vi "Read Debug Data Event.vi"(8 "error in (no error)":errorcluster, 11 "Debug Message Receiver In":refnum<class "Mock Debug Message Receiver.lvclass">) -> (0 "error out":errorcluster, 2 "Debug Data Event":refnum<user-event>, 3 "Debug Message Receiver Out":refnum<class "Mock Debug Message Receiver.lvclass">)   [LabVIEW 2020, in "Mock Debug Message Receiver.lvclass"]
uses:
  Mock Debug Message Receiver.lvclass
  Debug Message Receiver/Public/Debug Data Cluster.ctl
  Mock Debug Message Receiver.lvclass/Mock Debug Message Receiver.ctl
  Debug Data Event/Debug Data Event.lvclass
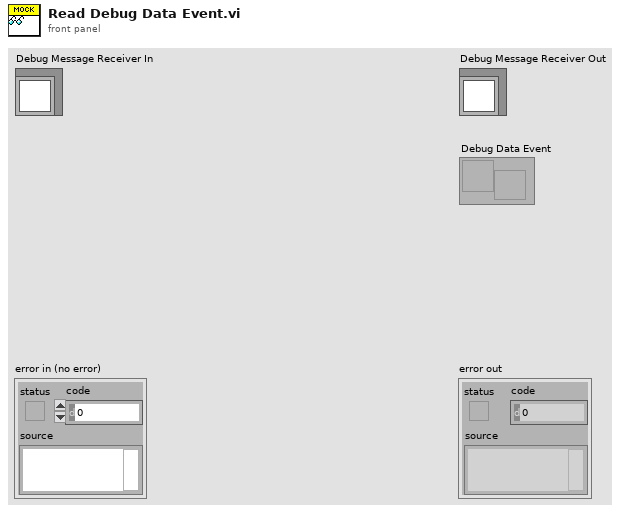
[diagram p1: front panel]
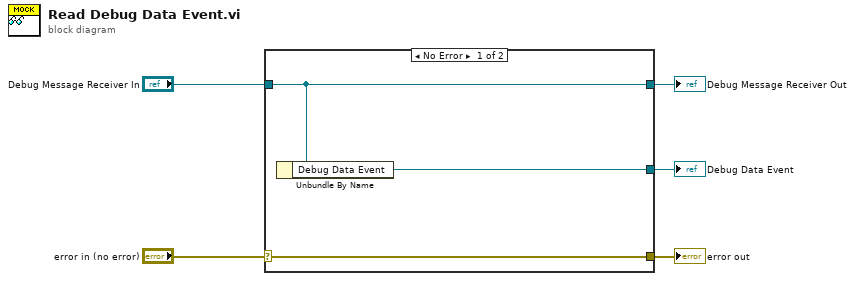
[diagram p0: block diagram]
diagram:
  n1 = case shown="No Error" "error in (no error)" {
    selector: "error in (no error)" -> [w8 w9]
    tunnel: [w8 w9] -> w4
    tunnel: [w7 w10] -> w2
    tunnel: "Debug Message Receiver In" -> [w7 w10]
    tunnel: [w6 _] -> w1
    frame No Error {
      n2 = Unbundle By Name(w7) -> ("Debug Data Event"=w6:refnum<user-event>)
    }
    frame Error {
    }
  }
  "error out" <- w4
  "Debug Message Receiver Out" <- w2
  "Debug Data Event" <- w1
